vi "LFA_AcquireWithAutosave.vi"(8 "error in (no error)":errorcluster, 11 "LightField Automation in":refnum<class "LightField Automation.lvclass">) -> (0 "error out":errorcluster, 2 "Data":T1(array[cluster]), 3 "LightField Automation out":refnum<class "LightField Automation.lvclass">)   [LabVIEW 2013, in "LightField Automation.lvclass"]
uses:
  LightField Automation.lvclass
  LightField Automation.lvclass/LightField Automation.ctl
  C:/Program Files/Princeton Instruments/LightField/AddInViews/PrincetonInstruments.LightFieldViewV3.dll
  Program Files/Princeton Instruments/LightField/AddInViews/PrincetonInstruments.LightFieldViewV3.dll
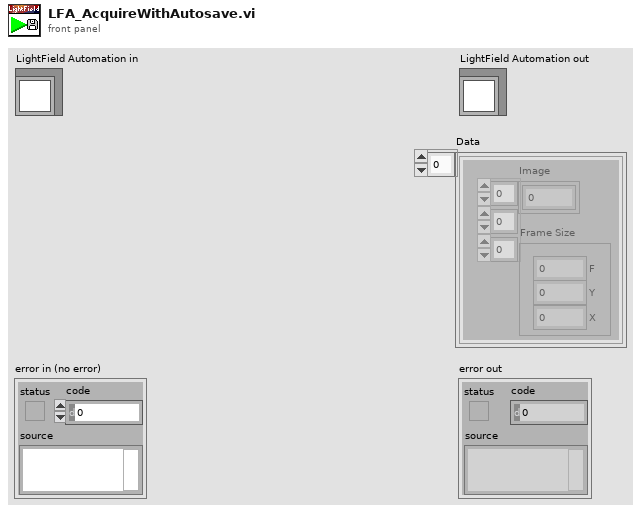
[diagram p1: front panel]
types:
  T1 = cluster{"Image":dbl[][][], "Frame Size":cluster{"F":i32, "Y":i32, "X":i32}}[]
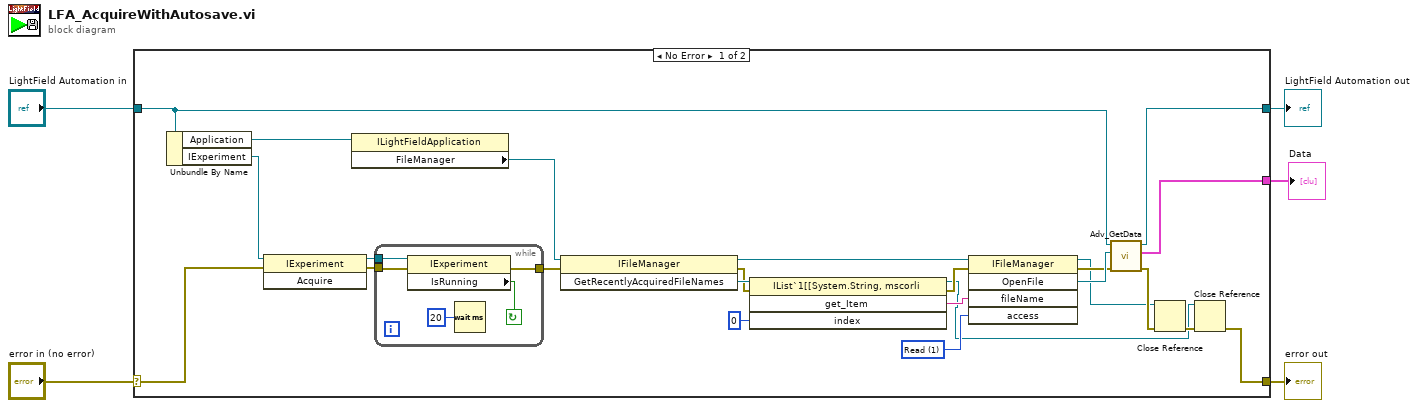
[diagram p0: block diagram]
diagram:
  n1 = case shown="No Error" "error in (no error)" {
    selector: "error in (no error)" -> [w29 w36]
    tunnel: [w7 w36] -> w4
    tunnel: [w25 w35] -> w2
    tunnel: "LightField Automation in" -> [w24 w35]
    tunnel: [w23 _] -> w1
    frame No Error {
      w13 = 1 items=["Read"=1, "Write"=2, "ReadWrite"=3] ("access")
      n2 = Unbundle By Name(w24) -> ("Application"=w22:refnum<k24>, "IExperiment"=w26:refnum<k24>)
      n3 = invoke class="IExperiment" method="Acquire"(reference=w26, error in=w29) -> (reference out=w27:refnum<k24>, error out=w28:errorcluster)  [unwired: 1 in, 1 out]
      n4 = property class="ILightFieldApplication"(reference=w22) -> ("FileManager"=w21:refnum<k24>)  [unwired: 1 in, 2 out]
      n5 = while {
        tunnel: w28 -> [w32]
        tunnel: [w31] -> w20
        tunnel: w27 -> [w30]
        stop <- w34 continue-if-true
        n6 = property class="IExperiment"(reference=w30, error in=w32) -> (error out=w31:errorcluster, "IsRunning"=w34:bool)  [unwired: 1 out]
        n7 = Wait (ms)(milliseconds to wait=u32 20) -> ()  [unwired: 1 out]
      }
      n8 = invoke class="IFileManager" method="GetRecentlyAcquiredFileNames"(reference=w21, error in=w20) -> (reference out=w15:refnum<k24>, error out=w18:errorcluster, "GetRecentlyAcquiredFileNames"=w19:refnum<k24>)  [unwired: 1 in]
      n9 = invoke class="IList`1[[System.String, mscorli" method="get_Item"(reference=w19, error in=w18, "index"=0) -> (reference out=w6:refnum<k24>, error out=w16:errorcluster, "get_Item"=w14:string)  [unwired: 1 in, 1 out]
      n10 = invoke class="IFileManager" method="OpenFile"(reference=w15, error in=w16, "fileName"=w14, "access"=w13) -> (reference out=w9:refnum<k24>, error out=w11:errorcluster, "OpenFile"=w12:refnum<k24>)  [unwired: 1 in, 2 out]
      n11 = call "Adv_GetData.vi"("error in (no error)"=w11, "IImageDataSet"=w12, "LightField Automation in"=w24) -> ("error out"=w10:errorcluster, "Data"=w23:T1, "LightField Automation out"=w25:refnum<class "LightField Automation.lvclass">)  [unwired: 6 in]
      n12 = Close Reference(reference=w9, error in (no error)=w10) -> (error out=w8:errorcluster)
      n13 = Close Reference(reference=w6, error in (no error)=w8) -> (error out=w7:errorcluster)
    }
    frame Error {
    }
  }
  "error out" <- w4
  "LightField Automation out" <- w2
  "Data" <- w1
